vi "Pause.vi"(8 "error in (no error)":errorcluster, 11 "Masterflex Settings in":T1={"VISA resource name"="", "Simulated?"=FALSE, "Pump Number"=1.0, "Reverse?"=FALSE} {"Pump Number" min=1.0 max=20.0 step=1.0}) -> (0 "error out":errorcluster, 1 "Connection Error":bool, 3 "Masterflex Settings out":T1={"VISA resource name"="", "Simulated?"=FALSE, "Pump Number"=1.0, "Reverse?"=FALSE} {"Pump Number" min=1.0 max=20.0 step=1.0})   [LabVIEW 2021, in "Masterflex 7550-30.lvlib"]
uses:
  Masterflex 7550-30.lvlib
  Controls/Settings Cluster.ctl
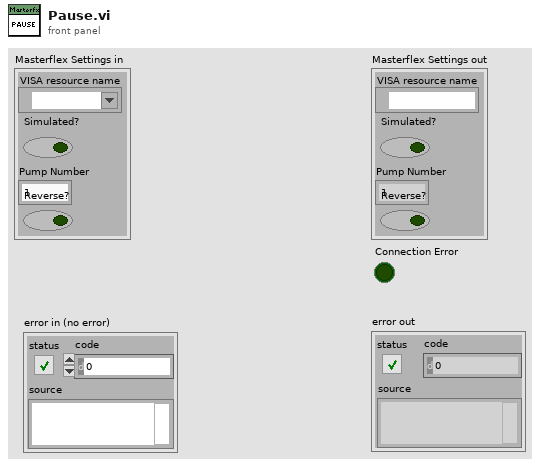
[diagram p1: front panel]
types:
  T1 = typedef "Masterflex 7550-30.lvlib/Settings Cluster.ctl" = cluster{"VISA resource name":refnum<visa-resource-name>, "Simulated?":bool, "Pump Number":dbl, "Reverse?":bool}
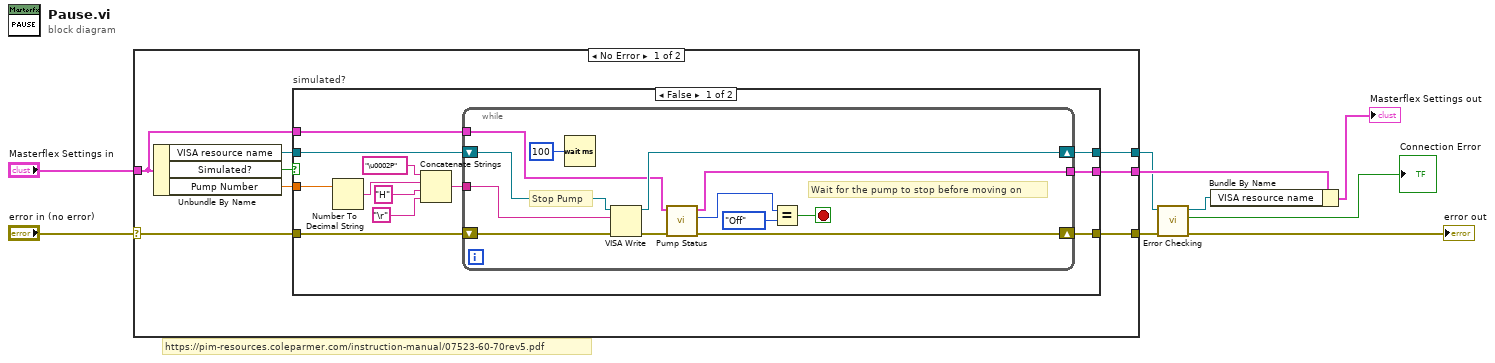
[diagram p0: block diagram]
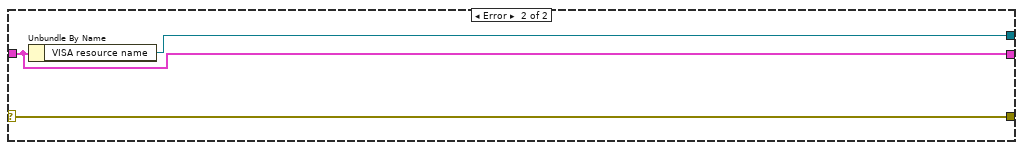
[diagram p3: hidden frame]
diagram:
  # "https://pim-resources.coleparmer.com/instruction-manual/07523-60-70rev5.pdf"
  n1 = case shown="No Error" "error in (no error)" {
    selector: "error in (no error)" -> [w15 w47]
    tunnel: [w11 w46] -> w9
    tunnel: "Masterflex Settings in" -> [w12 w46]
    tunnel: [w14 w45] -> w6
    tunnel: [w13 w47] -> w7
    frame No Error {
      n2 = Unbundle By Name(w12) -> ("VISA resource name"=w17:refnum<visa-resource-name>, "Simulated?"=w16:bool, "Pump Number"=w10:dbl)
      n3 = case "simulated?" shown="False" w16 {
        tunnel: [w27 w44] -> w14
        tunnel: w17 -> [w29 w44]
        tunnel: w15 -> [w28 w43]
        tunnel: [w26 w43] -> w13
        tunnel: w12 -> [w25 w42]
        tunnel: [w24 w42] -> w11
        tunnel: w10 -> [w22 _]
        frame False {
          n4 = Number To Decimal String(number=w22) -> (decimal integer string=w23:string)  [unwired: 1 in]
          n5 = Concatenate Strings("\u0002P" ("string"), w23, "H" ("string"), "\r") -> (w18:string)
          n6 = while {
            shift-right: [w39] -> w27
            shift-left: w29 -> [w41]
            shift-right: [w34] -> w26
            shift-left: w28 -> [w40]
            tunnel: w25 -> [w37]
            tunnel: [w36] -> w24
            tunnel: w18 -> [w30]
            stop <- w32 stop-if-true
            # "Wait for the pump to stop before moving on"
            # "Stop Pump"
            n7 = Wait (ms)(milliseconds to wait=u32 100) -> ()  [unwired: 1 out]
            n8 = VISA Write(VISA resource name=w41, write buffer=w30, error in (no error)=w40) -> (VISA resource name out=w39:refnum<visa-resource-name>, error out=w35:errorcluster)  [unwired: 1 out]
            n9 = call "Pump Status.vi"("error in (no error)"=w35, "Masterflex Settings in"=w37) -> ("error out"=w34:errorcluster, "Pump On?"=w33:enum16{"Off", "On", "Not Initialized"}, "Masterflex Settings out"=w36:T1)  [unwired: 6 in, 1 out]
            n10 = Equal?(x=w33, y=enum16{"Off", "On", "Not Initialized"}."Off") -> (x = y?=w32:bool)
          }
        }
        frame True {
        }
      }
    }
    frame Error {
      n11 = Unbundle By Name(w46) -> ("VISA resource name"=w45:refnum<visa-resource-name>)
    }
  }
  n12 = call "Error Checking.vi"("error in (no error)"=w7, "VISA resource name"=w6) -> ("error out"=→"error out":errorcluster, "Connection Error"=→"Connection Error":bool, "VISA resource name"=w8:refnum<visa-resource-name>)  [unwired: 7 in]
  n13 = Bundle By Name(cluster=w9, "VISA resource name"=w8) -> (→"Masterflex Settings out":T1)
